vi "IgniterTest.vi"() -> ()   [LabVIEW 2016]
panel:
  in  "Read From File":bool
  out "Numeric":dbl
  out "Waveform Chart":dynamicdata(graph)
  in  "stop (F)":bool
  in  "Ignite":bool
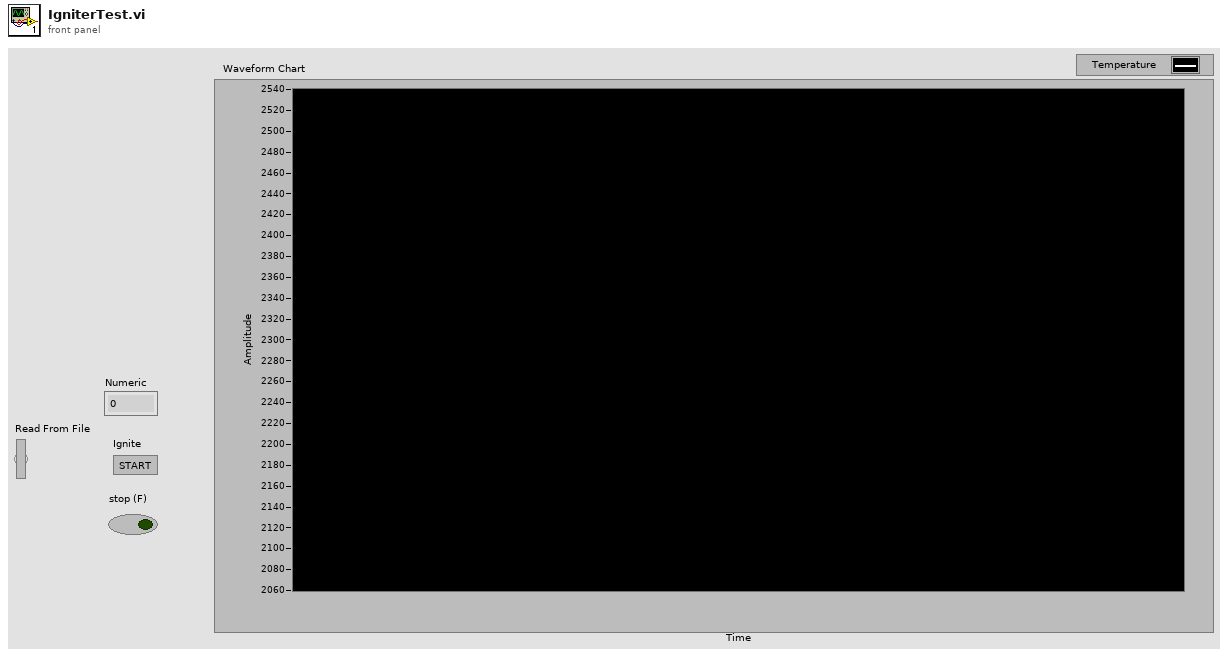
[diagram p1: front panel]
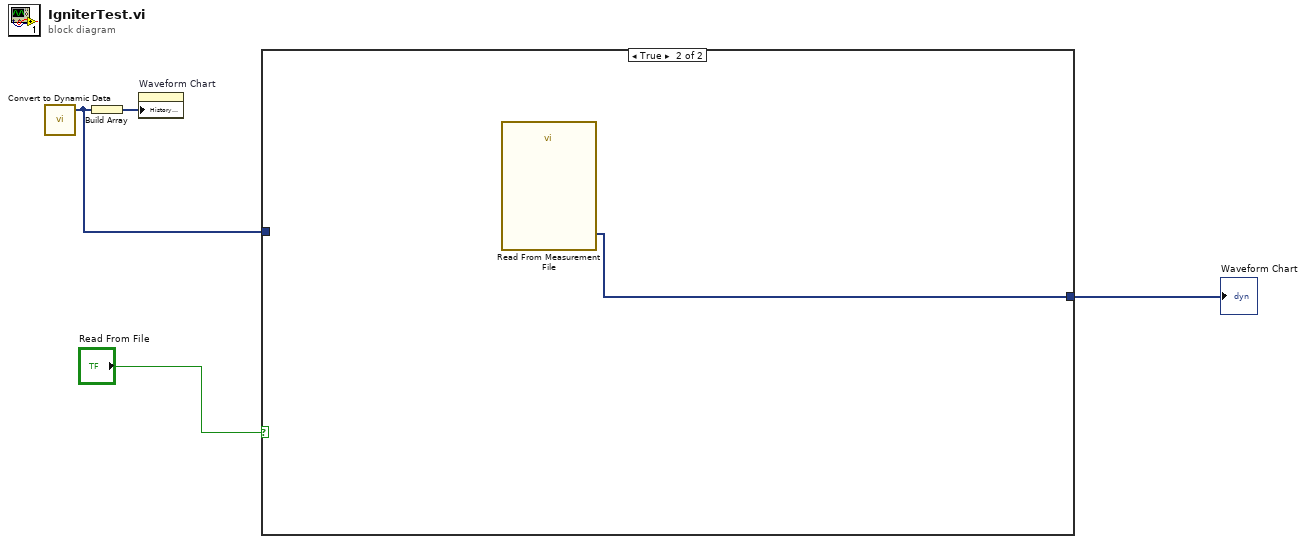
[diagram p0: block diagram]
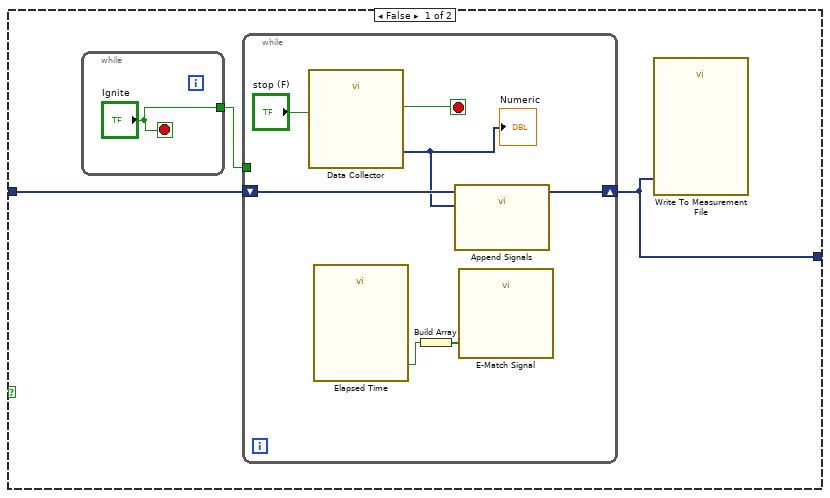
[diagram p2: hidden frame]
diagram:
  n1 = call "Convert to Dynamic Data"() -> ("Dynamic Data Type"=w2:dynamicdata)  [unwired: 4 in]
  n2 = Build Array(w2) -> (w3:dynamicdata[])
  n3 = property on="Waveform Chart" class="WFChart (strict)"("History Data"=w3) -> ()  [unwired: 2 in, 2 out]
  n4 = case shown="True" "Read From File" {
    tunnel: [w6 w16] -> w4
    tunnel: w2 -> [w5 _]
    frame False {
      n5 = while {
        tunnel: ["Ignite"] -> w7
        stop <- "Ignite" stop-if-true
      }
      n6 = while {
        shift-right: [w11] -> w6
        shift-left: w5 -> [w12]
        tunnel: w7 -> [_]
        stop <- w13 stop-if-true
        n7 = call "Data Collector"("stop (F)"="stop (F)") -> ("data"=w8:dynamicdata, "stopped"=w13:bool)  [unwired: 15 in, 2 out]
        "Numeric" <- w8
        n8 = call "Elapsed Time"() -> ("Time has Elapsed"=w10:bool)  [unwired: 12 in, 7 out]
        n9 = Build Array(w10) -> (w9:bool[])
        n10 = call "Append Signals"("Input Signal B"=w8, "Input Signal A"=w12) -> ("Appended Signals"=w11:dynamicdata)  [unwired: 8 in, 1 out]
        n11 = call "E-Match Signal"("data"=w9) -> ()  [unwired: 17 in, 2 out]
      }
      n12 = call "Write To Measurement File"("Signals"=w6) -> ()  [unwired: 16 in, 3 out]
    }
    frame True {
      n13 = call "Read From Measurement File"() -> ("Signals"=w16:dynamicdata)  [unwired: 6 in, 5 out]
    }
  }
  "Waveform Chart" <- w4
